vi "Create.vi"(10 "Status Tree":map{string[], T1}(c390)) -> (3 "StatusTreeValue out":refnum<class "StatusTreeValue.lvclass">)   [LabVIEW 2020, in "Volatus.lvlib" / "StatusTreeValue.lvclass"]
uses:
  StatusTreeValue.lvclass
  Module/State.ctl
  StatusTreeValue.lvclass/StatusTreeValue.ctl
  Module/Module.lvclass
  Module Status.ctl
  Volatus.lvlib
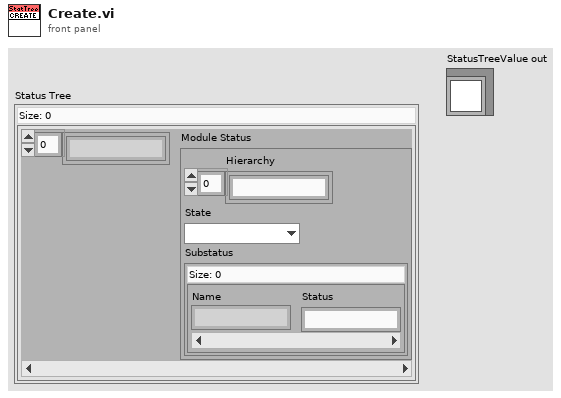
[diagram p1: front panel]
types:
  T1 = typedef "Volatus.lvlib/Module Status.ctl" = cluster{"Hierarchy":string[], "State":T2, "Substatus":map{string, string}}
  T2 = typedef "Volatus.lvlib/Module.lvclass/State.ctl" = enum16{"Unknown", "Launched", "Starting", "Running", "Stopping", "Stopped", "Error - Starting", "Error - Run", "Error - Stopping"}
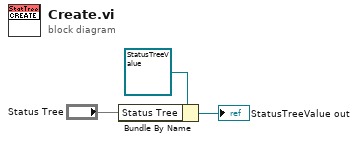
[diagram p0: block diagram]
diagram:
  n1 = Bundle By Name(cluster=refnum<class "StatusTreeValue.lvclass"> refnum ("StatusTreeValue out"), "Status Tree"="Status Tree") -> (→"StatusTreeValue out":refnum<class "StatusTreeValue.lvclass">)
